vi "NATS Server Start Windows.vi"(6 "Timeout (1000 ms)":i32=1000, 8 "error in":errorcluster, 9 "Monitor Port (8222)":i32=8222, 10 "Port (4222)":i32=4222, 11 "NATS Server EXE Path (default install)":path) -> (0 "error out":errorcluster, 3 "Active?":bool)   [LabVIEW 2020, in "NATS Infrastructure.lvlib"]
doc: "Stops NATS server on Windows machines."
uses:
  NATS Infrastructure.lvlib
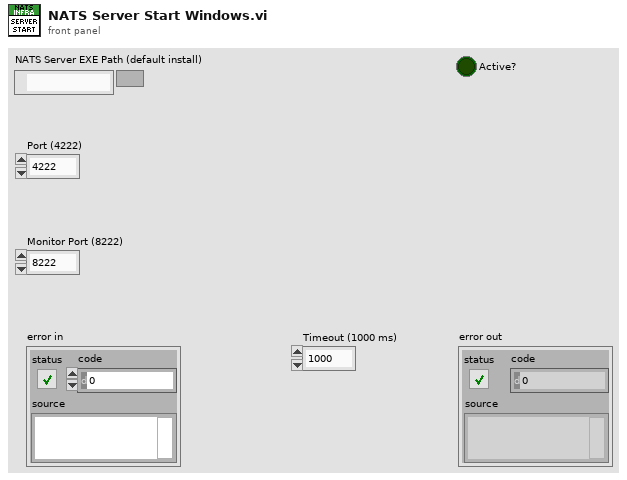
[diagram p1: front panel]
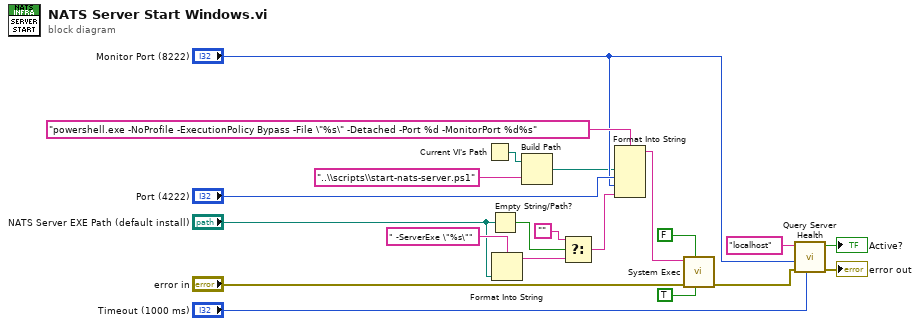
[diagram p0: block diagram]
diagram:
  n1 = Current VI's Path() -> (path=w8:path)
  n2 = Empty String/Path?(string/path="NATS Server EXE Path (default install)") -> (empty?=w4:bool)
  n3 = Format Into String(format string=" -ServerExe \"%s\"", "NATS Server EXE Path (default install)") -> (resulting string=w3:string)  [unwired: 2 in, 1 out]
  n4 = Build Path(base path=w8, name or relative path="..\\scripts\\start-nats-server.ps1") -> (appended path=w7:path)
  n5 = Select(t="", s=w4, f=w3) -> (s? t:f=w1:string)
  n6 = Format Into String(format string="powershell.exe -NoProfile -ExecutionPolicy Bypass -File \"%s\" -Detached -Port %d -MonitorPort %d%s" ("command line"), w7, "Port (4222)", "Monitor Port (8222)", w1) -> (resulting string=w16:string)  [unwired: 2 in, 1 out]
  n7 = call <vilib>:"System Exec.vi"("run minimized? (F)"=TRUE ("run minimized (T)"), "wait until completion? (T)"=FALSE, "error in (no error)"="error in", "command line"=w16) -> ("error out"=w11:errorcluster)  [unwired: 4 in, 3 out]
  n8 = call "Query Server Health.vi"("Timeout (1000 ms)"="Timeout (1000 ms)", "error in"=w11, "Monitor Port (8222)"="Monitor Port (8222)", "Server Address (localhost)"="localhost") -> ("error out"=→"error out":errorcluster, "healthy"=→"Active?":bool)  [unwired: 6 in]
